vi "CRYUnflatten Windows System.vi"(11 "Flatten WinSys":string) -> (0 "Error?":bool=TRUE, 2 "Windows System":T1, 3 "Header info":T3={"Data type"="Data            ", "Version"=1, "Dimensions"=0})   [LabVIEW 2013]
uses:
  Control/CRYWindows Sysem.ctl
  <vilib>/Utility/miscctls.llb/LVRectTypeDef.ctl
panel:
  out "ActiveWID=?":bool
  in  "nActiveWID":i32
  in  "nStepVINo":i32
  in  "sStepName":string
  out "FindStepFrame":bool
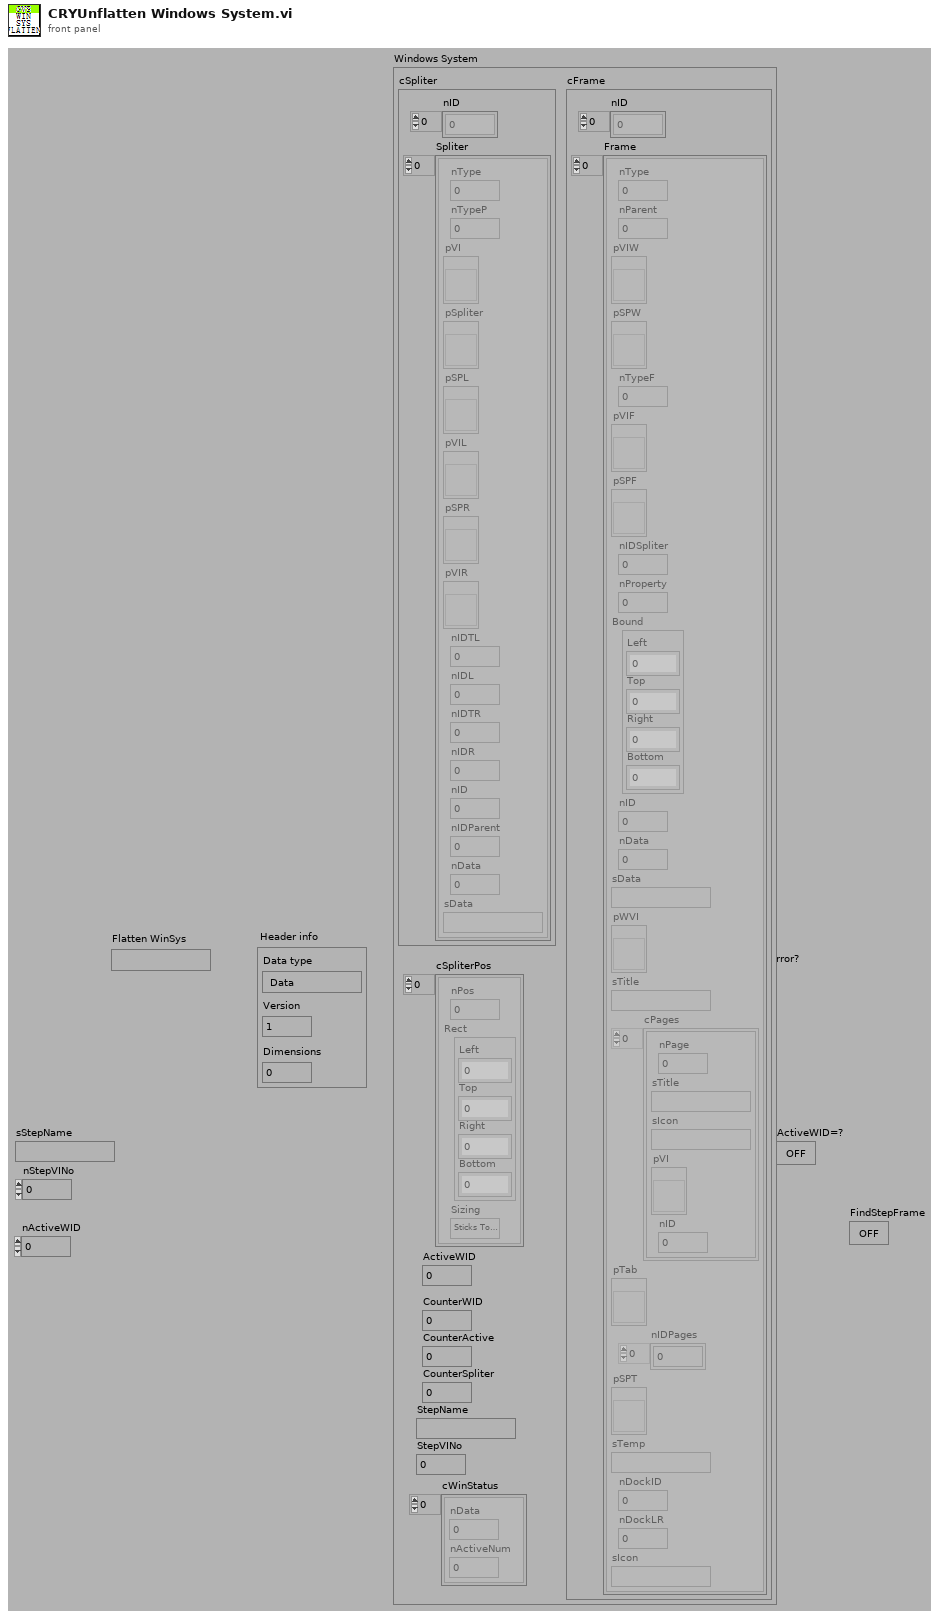
[diagram p1: front panel]
types:
  T1 = typedef "CRYWindows Sysem.ctl" = cluster{"cFrame":cluster{"nID":i32[], "Frame":cluster{"nType":i32, "nParent":i32, "pVIW":refnum<vi>, "pSPW":refnum<vi>, "nTypeF":i32, "pVIF":refnum<vi>, "pSPF":refnum<vi>, "nIDSpliter":i32, "nProperty":i32, "Bound":T2, "nID":i32, "nData":i32, "sData":string, "pWVI":refnum<vi>, "sTitle":string, "cPages":cluster{"nPage":i32, "sTitle":string, "sIcon":string, "pVI":refnum<vi>, "nID":i32}[], "pTab":refnum<vi>, "nIDPages":i32[], "pSPT":refnum<vi>, "sTemp":string, "nDockID":i32, "nDockLR":i32, "sIcon":string}[]}, "cSpliter":cluster{"nID":i32[], "Spliter":cluster{"nType":i32, "nTypeP":i32, "pVI":refnum<vi>, "pSpliter":refnum<vi>, "pSPL":refnum<vi>, "pVIL":refnum<vi>, "pSPR":refnum<vi>, "pVIR":refnum<vi>, "nIDTL":i32, "nIDL":i32, "nIDTR":i32, "nIDR":i32, "nID":i32, "nIDParent":i32, "nData":i32, "sData":string}[]}, "ActiveWID":i32, "cSpliterPos":cluster{"nPos":i32, "Rect":T2, "Sizing":enum16{"Sticks Top/Left", "Sticks Bottom/Right", "Proportional"}}[], "CounterWID":i32, "CounterActive":i32, "CounterSpliter":i32, "cWinStatus":cluster{"nData":i32, "nActiveNum":i32}[], "StepName":string, "StepVINo":i32}
  T2 = typedef "LVRectTypeDef.ctl" = cluster{"Left":i16, "Top":i16, "Right":i16, "Bottom":i16}
  T3 = cluster{"Data type":string, "Version":u16, "Dimensions":u8}
  T4 = cluster{"cFrame":cluster{"nID":i32[], "Frame":cluster{"nType":i32, "nParent":i32, "pVIW":refnum<vi>, "pSPW":refnum<vi>, "nTypeF":i32, "pVIF":refnum<vi>, "pSPF":refnum<vi>, "nIDSpliter":i32, "nProperty":i32, "Bound":T2, "nID":i32, "nData":i32, "sData":string, "pWVI":refnum<vi>, "sTitle":string, "cPages":cluster{"nPage":i32, "sTitle":string, "sIcon":string, "pVI":refnum<vi>, "nID":i32}[], "pTab":refnum<vi>, "nIDPages":i32[], "pSPT":refnum<vi>, "sTemp":string, "nDockID":i32, "nDockLR":i32, "sIcon":string}[]}, "cSpliter":cluster{"nID":i32[], "Spliter":cluster{"nType":i32, "nTypeP":i32, "pVI":refnum<vi>, "pSpliter":refnum<vi>, "pSPL":refnum<vi>, "pVIL":refnum<vi>, "pSPR":refnum<vi>, "pVIR":refnum<vi>, "nIDTL":i32, "nIDL":i32, "nIDTR":i32, "nIDR":i32, "nID":i32, "nIDParent":i32, "nData":i32, "sData":string}[]}, "ActiveWID":i32, "cSpliterPos":cluster{"nPos":i32, "Rect":T2, "Sizing":enum16{"Sticks Top/Left", "Sticks Bottom/Right", "Proportional"}}[], "CounterWID":i32, "CounterActive":i32, "CounterSpliter":i32, "cWinStatus":cluster{"nData":i32, "nActiveNum":i32}[], "StepName":string, "StepVINo":i32}
  T5 = cluster{"nType":i32, "nParent":i32, "pVIW":refnum<vi>, "pSPW":refnum<vi>, "nTypeF":i32, "pVIF":refnum<vi>, "pSPF":refnum<vi>, "nIDSpliter":i32, "nProperty":i32, "Bound":T2, "nID":i32, "nData":i32, "sData":string, "pWVI":refnum<vi>, "sTitle":string, "cPages":cluster{"nPage":i32, "sTitle":string, "sIcon":string, "pVI":refnum<vi>, "nID":i32}[], "pTab":refnum<vi>, "nIDPages":i32[], "pSPT":refnum<vi>, "sTemp":string, "nDockID":i32, "nDockLR":i32, "sIcon":string}[]
  T6 = cluster{"nPage":i32, "sTitle":string, "sIcon":string, "pVI":refnum<vi>, "nID":i32}[]
  T7 = cluster{"unsigned byte array[0]":u8, "unsigned byte array[1]":u8, "unsigned byte array[2]":u8}
  T8 = cluster{"cFrame":cluster{"nID":i32[], "Frame":cluster{"nType":i32, "nParent":i32, "pVIW":refnum<vi>, "pSPW":refnum<vi>, "nTypeF":i32, "pVIF":refnum<vi>, "pSPF":refnum<vi>, "nIDSpliter":i32, "nProperty":i32, "Bound":T2, "nID":i32, "nData":i32, "sData":string, "pWVI":refnum<vi>, "sTitle":string, "cPages":cluster{"nPage":i32, "sTitle":string, "sIcon":string, "pVI":refnum<vi>, "nID":i32}[], "pTab":refnum<vi>, "nIDPages":i32[], "pSPT":refnum<vi>, "sTemp":string, "nDockID":i32, "nDockLR":i32, "sIcon":string}[]}, "cSpliter":cluster{"nID":i32[], "Spliter":cluster{"nType":i32, "nTypeP":i32, "pVI":refnum<vi>, "pSpliter":refnum<vi>, "pSPL":refnum<vi>, "pVIL":refnum<vi>, "pSPR":refnum<vi>, "pVIR":refnum<vi>, "nIDTL":i32, "nIDL":i32, "nIDTR":i32, "nIDR":i32, "nID":i32, "nIDParent":i32, "nData":i32, "sData":string}[]}, "ActiveWID":i32, "cSpliterPos":cluster{"nPos":i32, "Rect":T2, "Sizing":enum16{"Sticks Top/Left", "Sticks Bottom/Right", "Proportional"}}[], "CounterWID":i32, "CounterActive":i32, "CounterSpliter":i32, "cWinStatus":cluster{"nData":i32, "nActiveNum":i32}[], "sWsysVersion":string}
  T9 = cluster{"nID":i32[], "Frame":cluster{"nType":i32, "nParent":i32, "pVIW":refnum<vi>, "pSPW":refnum<vi>, "nTypeF":i32, "pVIF":refnum<vi>, "pSPF":refnum<vi>, "nIDSpliter":i32, "nProperty":i32, "Bound":T2, "nID":i32, "nData":i32, "sData":string, "pWVI":refnum<vi>, "sTitle":string, "cPages":cluster{"nPage":i32, "sTitle":string, "sIcon":string, "pVI":refnum<vi>, "nID":i32}[], "pTab":refnum<vi>, "nIDPages":i32[], "pSPT":refnum<vi>, "sTemp":string, "nDockID":i32, "nDockLR":i32, "sIcon":string}[]}
  T10 = cluster{"nID":i32[], "Spliter":cluster{"nType":i32, "nTypeP":i32, "pVI":refnum<vi>, "pSpliter":refnum<vi>, "pSPL":refnum<vi>, "pVIL":refnum<vi>, "pSPR":refnum<vi>, "pVIR":refnum<vi>, "nIDTL":i32, "nIDL":i32, "nIDTR":i32, "nIDR":i32, "nID":i32, "nIDParent":i32, "nData":i32, "sData":string}[]}
  T11 = cluster{"nPos":i32, "Rect":T2, "Sizing":enum16{"Sticks Top/Left", "Sticks Bottom/Right", "Proportional"}}[]
  T12 = cluster{"sStepName":string, "nStepVINo":i32, "nStepVINoDisplay":i32}
  T13 = cluster{"nType":i32, "nParent":i32, "pVIW":refnum<vi>, "pSPW":refnum<vi>, "nTypeF":i32, "pVIF":refnum<vi>, "pSPF":refnum<vi>, "nIDSpliter":i32, "nProperty":i32, "Bound":T2, "nID":i32, "nData":i32, "sData":string, "pWVI":refnum<vi>, "sTitle":string, "cPages":cluster{"nPage":i32, "sTitle":string, "sIcon":string, "pVI":refnum<vi>, "nID":i32}[], "pTab":refnum<vi>, "nIDPages":i32[], "pSPT":refnum<vi>, "sTemp":string, "nDockID":i32, "nDockLR":i32, "sIcon":string}
  T14 = cluster{"substring":string, u16, "unsigned byte array[2]":u8}
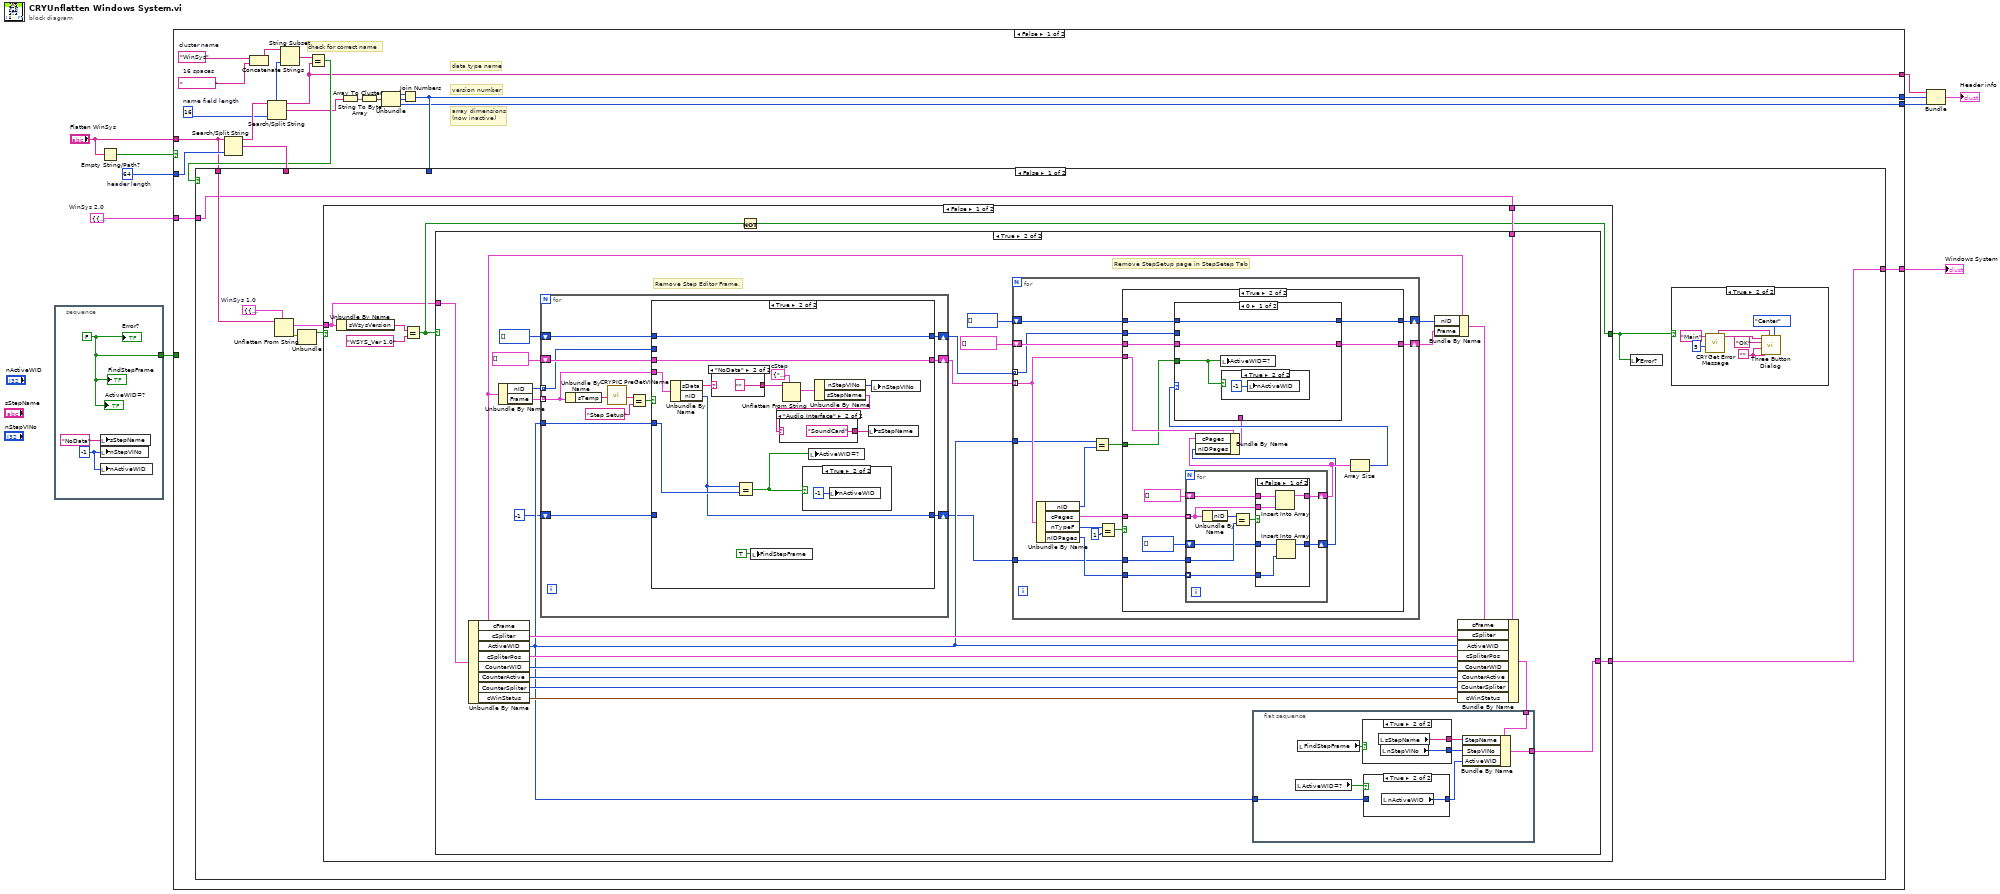
[diagram p0: block diagram]
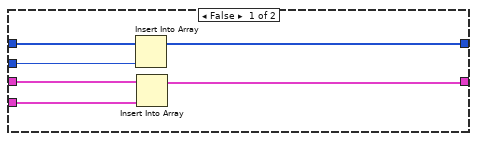
[diagram p4: hidden frame]
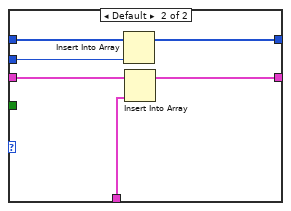
[diagram p6: hidden frame]
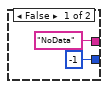
[diagram p9: hidden frame]
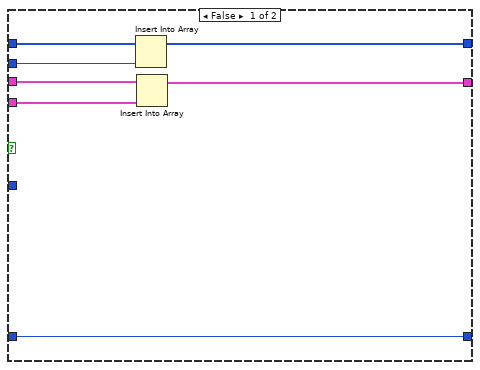
[diagram p10: hidden frame]
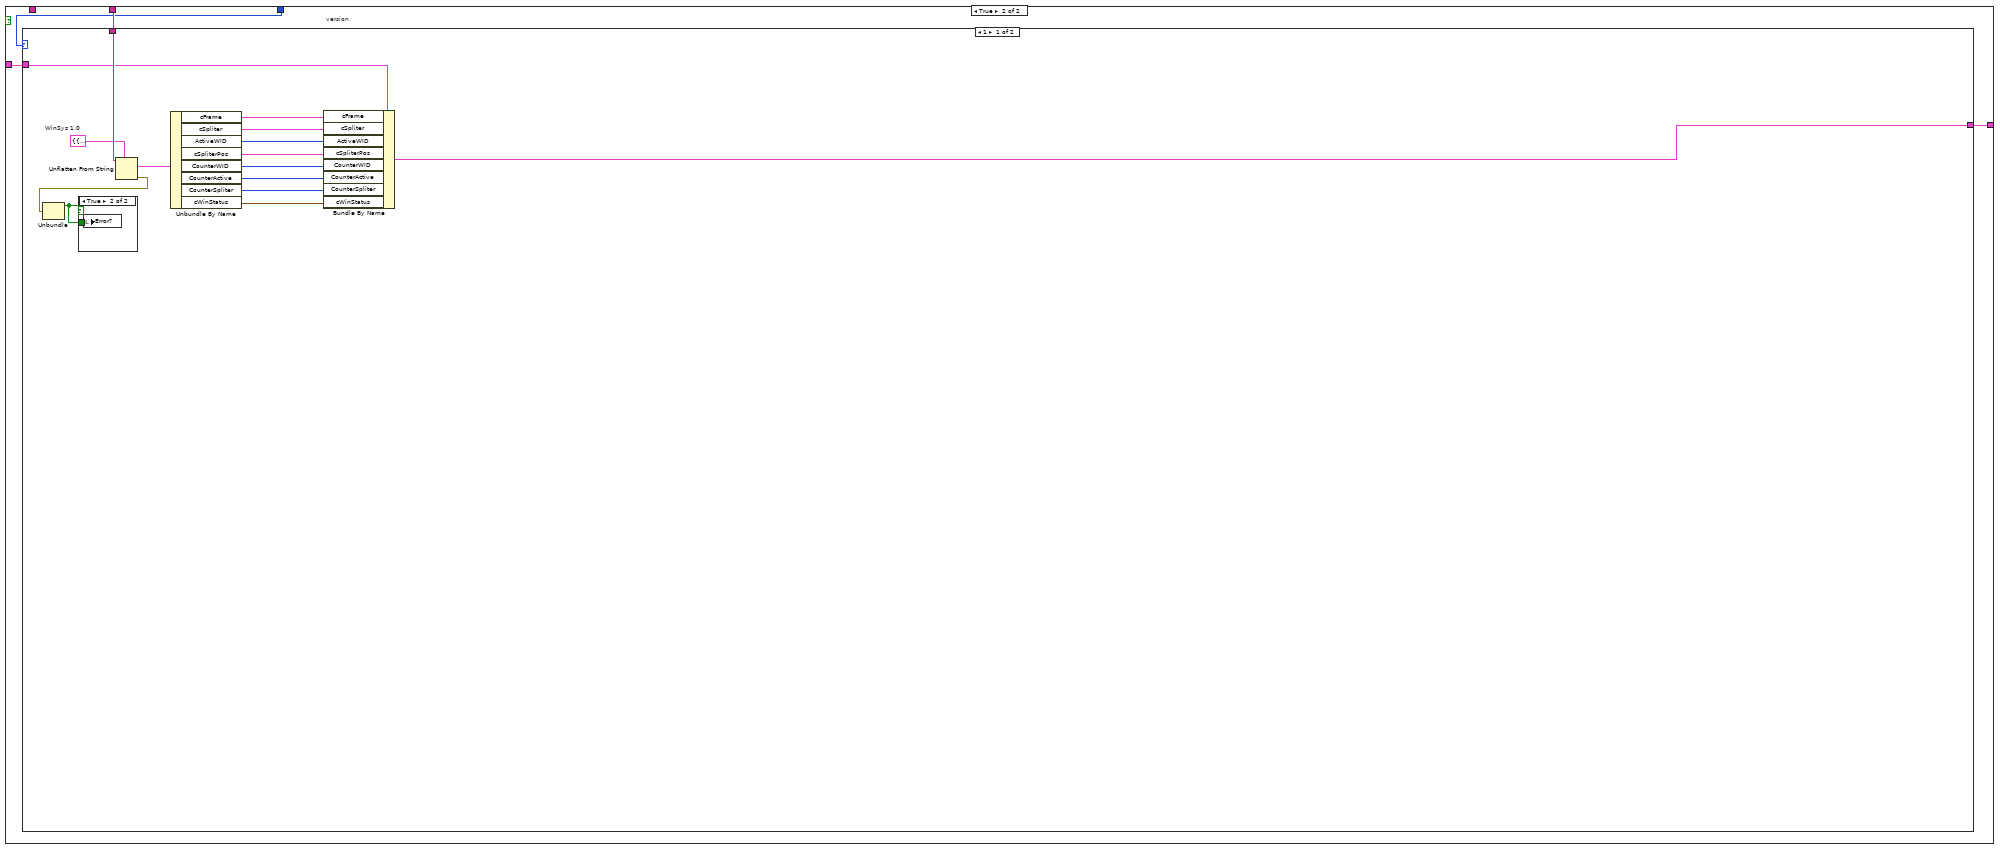
[diagram p15: hidden frame]
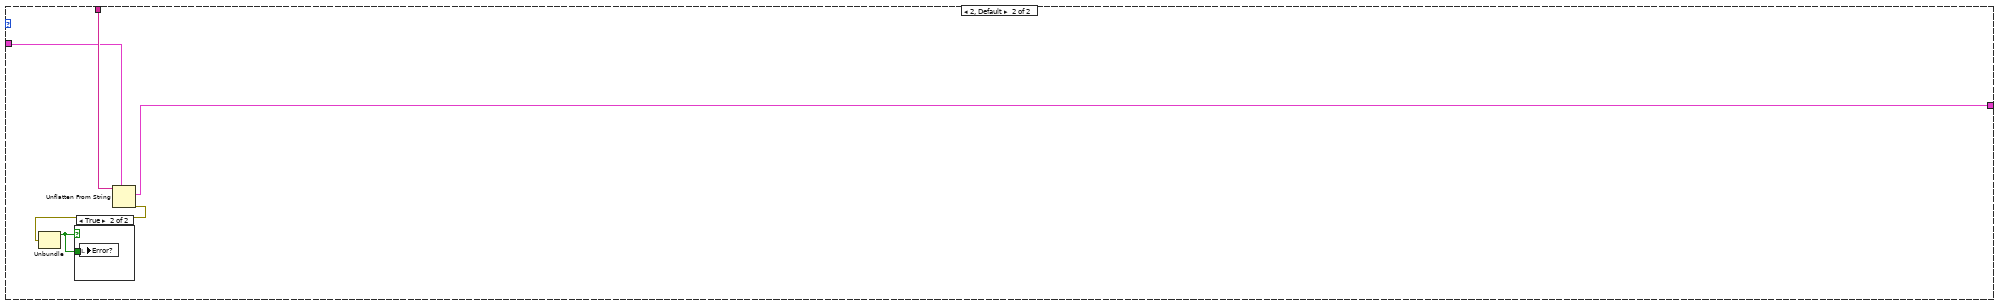
[diagram p17: hidden frame]
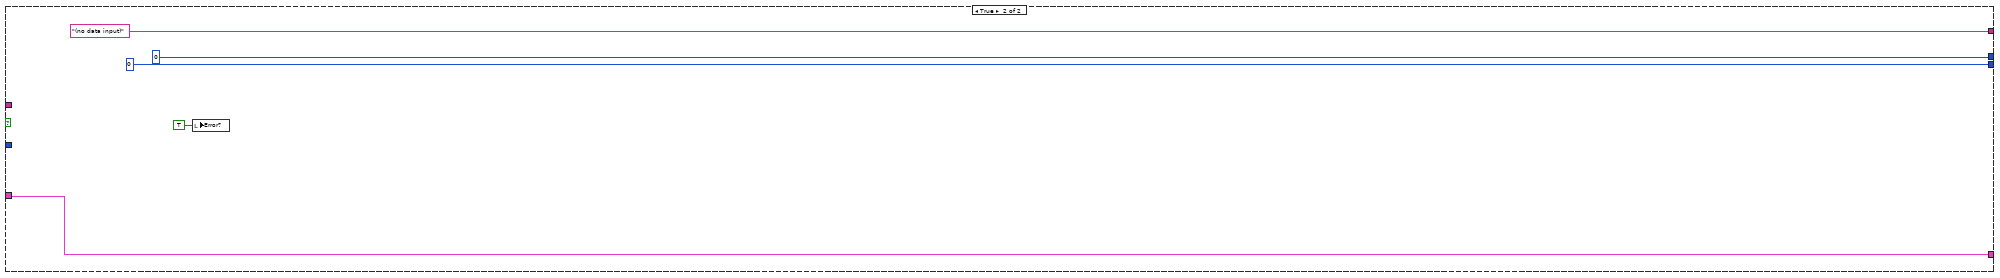
[diagram p19: hidden frame]
diagram:
  w2 = T4 {"cFrame"={"nID"=[], "Frame"=[]}, "cSpliter"={"nID"=[], "Spliter"=[]}, "ActiveWID"=0, "cSpliterPos"=[], "CounterWID"=0, "CounterActive"=0, "CounterSpliter"=0, "cWinStatus"=[], "StepName"="", "StepVINo"=0}  # WinSys 2.0
  w8 = 64  # header length
  n1 = stacked-sequence {
    tunnel: [w12] -> w3
    frame #0 {
      w11 = -1 ("nStepVINo")
      w12 = FALSE
      n2 = local write "sStepName"("NoData" ("sStepName")) -> ()
      n3 = local write "nStepVINo"(w11) -> ()
      n4 = local write "nActiveWID"(w11) -> ()
      "Error?" <- w12
      "FindStepFrame" <- w12
      "ActiveWID=?" <- w12
    }
  }
  n5 = Empty String/Path?(string/path="Flatten WinSys") -> (empty?=w9:bool)
  n6 = case shown="False" w9 {
    tunnel: "Flatten WinSys" -> [w14 _]
    tunnel: w8 -> [w28 _]
    tunnel: [w25 u16 0] -> w6
    tunnel: [w17 u8 0] -> w7
    tunnel: [w18 "(no data input)" ("substring")] -> w5
    tunnel: w3 -> [_ _]
    tunnel: [w16 w227] -> w1
    tunnel: w2 -> [w15 w227]
    frame False {
      w22 = "                "  # 16 spaces
      w23 = "WinSys"  # cluster name
      w20 = 16  # name field length
      # "check for correct name"
      # "array dimensions\n(now inactive)"
      # "version number"
      # "data type name"
      n7 = Search/Split String(string=w14, offset (0)=w28) -> (substring before match=w27:string, match + rest of string=w29:string)  [unwired: 2 out]
      n8 = Concatenate Strings(w23, w22) -> (w21:string)
      n9 = Search/Split String(string=w27, offset (0)=w20) -> (substring before match=w18:string, match + rest of string=w24:string)  [unwired: 2 out]
      n10 = String Subset(string=w21, length (rest)=w20) -> (substring=w19:string)  [unwired: 1 out]
      n11 = Equal?(x=w19, y=w18) -> (x = y?=w26:bool)
      n12 = String To Byte Array(string=w24) -> (unsigned byte array=w33:u8[])
      n13 = Array To Cluster(array=w33) -> (cluster=w32:T7)
      n14 = Unbundle(w32) -> ("unsigned byte array[0]"=w31:u8, "unsigned byte array[1]"=w30:u8, "unsigned byte array[2]"=w17:u8)
      n15 = Join Numbers(hi=w31, lo=w30) -> ((hi.lo)=w25:u16)
      n16 = case shown="False" w26 {
        tunnel: w29 -> [_ w204]
        tunnel: w25 -> [_ w203]
        tunnel: [w35 w202] -> w16
        tunnel: w15 -> [w36 w201]
        tunnel: w14 -> [w40 _]
        frame False {
          w34 = T8 {"cFrame"={"nID"=[], "Frame"=[]}, "cSpliter"={"nID"=[], "Spliter"=[]}, "ActiveWID"=0, "cSpliterPos"=[], "CounterWID"=0, "CounterActive"=0, "CounterSpliter"=0, "cWinStatus"=[], "sWsysVersion"=""}  # WinSys 1.0
          n17 = Unflatten From String(type=w34, binary string=w40) -> (value=w41:T8, error out=w39:errorcluster)  [unwired: 1 in, 3 out]
          n18 = Unbundle(w39) -> ("status"=w38:bool)  [unwired: 2 out]
          n19 = case shown="False" w38 {
            selector: w38 -> [_ w200]
            tunnel: w41 -> [w52 _]
            tunnel: [w49 w200] -> w37
            tunnel: w36 -> [w51 w199]
            tunnel: [w50 w199] -> w35
            frame False {
              n20 = Unbundle By Name(w52) -> ("sWsysVersion"=w55:string)
              n21 = Equal?(x=w55, y="WSYS_Ver 1.0" ("sWsysVersion")) -> (x = y?=w53:bool)
              n22 = case shown="True" w53 {
                tunnel: w52 -> [_ w75]
                tunnel: w51 -> [w56 w74]
                tunnel: [w56 w60] -> w50
                frame False {
                }
                frame True {
                  # "Remove StepSetup page in StepSetep Tab"
                  # "Remove Step Editor Frame."
                  n23 = Unbundle By Name(w75) -> ("cFrame"=w63:T9, "cSpliter"=w76:T10, "ActiveWID"=w59:i32, "cSpliterPos"=w77:T11, "CounterWID"=w78:i32, "CounterActive"=w79:i32, "CounterSpliter"=w80:i32, "cWinStatus"=w81:cluster{"nData":i32, "nActiveNum":i32}[])
                  n24 = Unbundle By Name(w63) -> ("nID"=w71:i32[], "Frame"=w73:T5)
                  n25 = for {
                    tunnel: w73 -> [w163] mode=indexing
                    shift-right: [w168] -> w66
                    shift-left: T5 [] ("Frame") -> [w169]
                    tunnel: w71 -> [w165] mode=indexing
                    shift-right: [w166] -> w67
                    shift-left: i32[] [] ("nID") -> [w167]
                    tunnel: w59 -> [w162]
                    shift-right: [w160] -> w57
                    shift-left: -1 ("ActiveWID") -> [w161]
                    n26 = Unbundle By Name(w163) -> ("sTemp"=w172:string)
                    n27 = call "CRYPIC PreGetVIName.vi"("sVIName"=w172) -> ("sVIName_Out"=w170:string)  [unwired: 9 in, 1 out]
                    n28 = Equal?(x=w170, y="Step Setup" ("sWsysVersion")) -> (x = y?=w164:bool)
                    n29 = case shown="True" w164 {
                      tunnel: w169 -> [w179 w192]
                      tunnel: [w178 w192] -> w168
                      tunnel: w163 -> [w177 w190]
                      tunnel: w167 -> [w176 w193]
                      tunnel: [w175 w193] -> w166
                      tunnel: w165 -> [w174 _]
                      tunnel: w162 -> [_ w184]
                      tunnel: w161 -> [w173 _]
                      tunnel: [w173 w182] -> w160
                      frame False {
                        n30 = Insert Into Array(array=w176, new element=w174) -> (w175:i32[])  [unwired: 1 in]
                        n31 = Insert Into Array(array=w179, new element=w177) -> (w178:T5)  [unwired: 1 in]
                      }
                      frame True {
                        w187 = T12 {"sStepName"="", "nStepVINo"=0, "nStepVINoDisplay"=0}  # cStep
                        n32 = Unbundle By Name(w190) -> ("sData"=w189:string, "nID"=w182:i32)
                        n33 = case shown="\"NoData\"" w189 {
                          selector: w189 -> [w197 _]
                          tunnel: [w197 "" ("sData")] -> w191
                          frame Default {
                          }
                          frame "NoData" {
                          }
                        }
                        n34 = Equal?(x=w182, y=w184) -> (x = y?=w183:bool)
                        n35 = local write "FindStepFrame"(TRUE ("Version=1?")) -> ()
                        n36 = Unflatten From String(type=w187, binary string=w191) -> (value=w186:T12)  [unwired: 1 in, 4 out]
                        n37 = case shown="True" w183 {
                          frame False {
                          }
                          frame True {
                            n38 = local write "nActiveWID"(-1 ("nActiveWID")) -> ()
                          }
                        }
                        n39 = local write "ActiveWID=?"(w183) -> ()
                        n40 = Unbundle By Name(w186) -> ("nStepVINo"=w185:i32, "sStepName"=w181:string)
                        n41 = case shown="\"Audio Interface\"" w181 {
                          selector: w181 -> [w194 _]
                          tunnel: [w194 "SoundCard"] -> w180
                          frame Default {
                          }
                          frame "Audio Interface" {
                          }
                        }
                        n42 = local write "sStepName"(w180) -> ()
                        n43 = local write "nStepVINo"(w185) -> ()
                      }
                    }
                  }
                  n44 = for {
                    tunnel: w66 -> [w88] mode=indexing
                    shift-right: [w95] -> w64
                    shift-left: T5 [] ("Frame") -> [w96]
                    tunnel: w67 -> [w92] mode=indexing
                    shift-right: [w93] -> w65
                    shift-left: i32[] [] ("nID") -> [w94]
                    tunnel: w57 -> [w85]
                    tunnel: w59 -> [w83]
                    n45 = Unbundle By Name(w88) -> ("nID"=w84:i32, "cPages"=w87:T6, "nTypeF"=w91:i32, "nIDPages"=w86:i32[])
                    n46 = Equal?(x=w83, y=w84) -> (x = y?=w82:bool)
                    n47 = Equal?(x=w91, y=1) -> (x = y?=w89:bool)
                    n48 = case shown="True" w89 {
                      tunnel: w96 -> [w102 w115]
                      tunnel: [w101 w112] -> w95
                      tunnel: w88 -> [w100 w110]
                      tunnel: w94 -> [w99 w114]
                      tunnel: [w98 w113] -> w93
                      tunnel: w92 -> [w97 w108]
                      tunnel: w87 -> [_ w111]
                      tunnel: w85 -> [_ w117]
                      tunnel: w86 -> [_ w105]
                      tunnel: w82 -> [_ w103]
                      frame False {
                        n49 = Insert Into Array(array=w99, new element=w97) -> (w98:i32[])  [unwired: 1 in]
                        n50 = Insert Into Array(array=w102, new element=w100) -> (w101:T5)  [unwired: 1 in]
                      }
                      frame True {
                        n51 = for {
                          tunnel: w111 -> [w132] mode=indexing
                          shift-right: [w133] -> w109
                          shift-left: T6 [] ("cPages") -> [w136]
                          tunnel: w117 -> [w134]
                          shift-right: [w130] -> w104
                          shift-left: i32[] [] ("nIDPages") -> [w131]
                          tunnel: w105 -> [w129] mode=indexing
                          n52 = Unbundle By Name(w132) -> ("nID"=w137:i32)
                          n53 = Equal?(x=w137, y=w134) -> (x = y?=w135:bool)
                          n54 = case shown="False" w135 {
                            tunnel: w136 -> [w143 w145]
                            tunnel: [w142 w145] -> w133
                            tunnel: w132 -> [w141 _]
                            tunnel: w131 -> [w140 w144]
                            tunnel: [w139 w144] -> w130
                            tunnel: w129 -> [w138 _]
                            frame False {
                              n55 = Insert Into Array(array=w143, new element=w141) -> (w142:T6)  [unwired: 1 in]
                              n56 = Insert Into Array(array=w140, new element=w138) -> (w139:i32[])  [unwired: 1 in]
                            }
                            frame True {
                            }
                          }
                        }
                        n57 = Bundle By Name(cluster=w110, "cPages"=w109, "nIDPages"=w104) -> (w107:T13)
                        n58 = Array Size(array=w109) -> (size(s)=w116:i32)
                        n59 = case shown="0" w116 {
                          tunnel: w115 -> [w120 w125]
                          tunnel: w114 -> [w121 w128]
                          tunnel: [w121 w126] -> w113
                          tunnel: [w120 w124] -> w112
                          tunnel: w108 -> [_ w127]
                          tunnel: w107 -> [_ w123]
                          tunnel: w103 -> [w119 _]
                          frame 0 {
                            n60 = local write "ActiveWID=?"(w119) -> ()
                            n61 = case shown="True" w119 {
                              frame False {
                              }
                              frame True {
                                n62 = local write "nActiveWID"(-1 ("nActiveWID")) -> ()
                              }
                            }
                          }
                          frame Default {
                            n63 = Insert Into Array(array=w128, new element=w127) -> (w126:i32[])  [unwired: 1 in]
                            n64 = Insert Into Array(array=w125, new element=w123) -> (w124:T5)  [unwired: 1 in]
                          }
                        }
                      }
                    }
                  }
                  n65 = flat-sequence {
                    tunnel: w61 -> [w152]
                    tunnel: w59 -> [w148]
                    tunnel: [w146] -> w60
                    frame #0 {
                      n66 = local read "ActiveWID=?"() -> (w149:bool)
                      n67 = local read "FindStepFrame"() -> (w153:bool)
                      n68 = case shown="True" w153 {
                        tunnel: ["NoData" ("sStepName") w159] -> w151
                        tunnel: [-1 ("nStepVINo") w158] -> w150
                        frame False {
                        }
                        frame True {
                          n69 = local read "sStepName"() -> (w159:string)
                          n70 = local read "nStepVINo"() -> (w158:i32)
                        }
                      }
                      n71 = case shown="True" w149 {
                        tunnel: [w154 w155] -> w147
                        tunnel: w148 -> [w154 _]
                        frame False {
                        }
                        frame True {
                          n72 = local read "nActiveWID"() -> (w155:i32)
                        }
                      }
                      n73 = Bundle By Name(cluster=w152, "StepName"=w151, "StepVINo"=w150, "ActiveWID"=w147) -> (w146:T4)
                    }
                  }
                  n74 = Bundle By Name(cluster=w63, "nID"=w65, "Frame"=w64) -> (w62:T9)
                  n75 = Bundle By Name(cluster=w74, "cFrame"=w62, "cSpliter"=w76, "ActiveWID"=w59, "cSpliterPos"=w77, "CounterWID"=w78, "CounterActive"=w79, "CounterSpliter"=w80, "cWinStatus"=w81) -> (w61:T4)
                }
              }
              n76 = Not(x=w53) -> (.not. x?=w49:bool)
            }
            frame True {
            }
          }
          n77 = local write "Error?"(w37) -> ()
          n78 = case shown="True" w37 {
            frame False {
            }
            frame True {
              w48 = ""
              n79 = call "CRYGet Error Message.vi"("Error No"=5, "Kind"="Main") -> ("Message"=w43:string, "Window Title"=w42:string)  [unwired: 4 in, 4 out]
              n80 = call <vilib>:"Three Button Dialog.vi"("Justify Message (Left)"=enum16{"Left", "Center", "Right"}."Center", "Window Title (\"\")"=w42, "Right Button Text (\"Cancel\")"=w48, "Center Button Text (\"No\")"=w48, "Left Button Text (\"Yes\")"="OK" ("Left Button Text (\"Yes\")"), "message"=w43) -> ()  [unwired: 6 out]
            }
          }
        }
        frame True {
          n81 = case "version" shown="1" w203 {
            tunnel: w204 -> [w219 w225]
            tunnel: [w216 w222] -> w202
            tunnel: w201 -> [w215 w221]
            frame 1 {
              w214 = T8 {"cFrame"={"nID"=[], "Frame"=[]}, "cSpliter"={"nID"=[], "Spliter"=[]}, "ActiveWID"=0, "cSpliterPos"=[], "CounterWID"=0, "CounterActive"=0, "CounterSpliter"=0, "cWinStatus"=[], "sWsysVersion"=""}  # WinSys 1.0
              n82 = Unflatten From String(type=w214, binary string=w219) -> (value=w213:T8, error out=w217:errorcluster)  [unwired: 1 in, 3 out]
              n83 = Unbundle(w217) -> ("status"=w218:bool)  [unwired: 2 out]
              n84 = case shown="True" w218 {
                tunnel: w218 -> [_ w220]
                frame False {
                }
                frame True {
                  n85 = local write "Error?"(w220) -> ()
                }
              }
              n86 = Unbundle By Name(w213) -> ("cFrame"=w212:T9, "cSpliter"=w211:T10, "ActiveWID"=w210:i32, "cSpliterPos"=w209:T11, "CounterWID"=w208:i32, "CounterActive"=w207:i32, "CounterSpliter"=w206:i32, "cWinStatus"=w205:cluster{"nData":i32, "nActiveNum":i32}[])
              n87 = Bundle By Name(cluster=w215, "cFrame"=w212, "cSpliter"=w211, "ActiveWID"=w210, "cSpliterPos"=w209, "CounterWID"=w208, "CounterActive"=w207, "CounterSpliter"=w206, "cWinStatus"=w205) -> (w216:T4)
            }
            frame 2, Default {
              n88 = Unflatten From String(type=w221, binary string=w225) -> (value=w222:T4, error out=w223:errorcluster)  [unwired: 1 in, 3 out]
              n89 = Unbundle(w223) -> ("status"=w224:bool)  [unwired: 2 out]
              n90 = case shown="True" w224 {
                tunnel: w224 -> [_ w226]
                frame False {
                }
                frame True {
                  n91 = local write "Error?"(w226) -> ()
                }
              }
            }
          }
        }
      }
    }
    frame True {
      n92 = local write "Error?"(TRUE ("Error?")) -> ()
    }
  }
  "Windows System" <- w1
  n93 = Bundle("substring"=w5, w6, "unsigned byte array[2]"=w7) -> (→"Header info":T14)  [unwired: 1 out]
